vi "Acq FOR loop exit logic.vi"(8 "error in (no error)":errorcluster) -> (0 "error out (dupl)":errorcluster, 3 "Stop acquisition FOR loop":bool)   [LabVIEW 2013]
uses:
  Typedefs/Read Write Enum.ctl
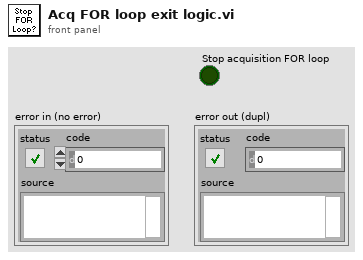
[diagram p1: front panel]
types:
  T1 = typedef "Read Write Enum.ctl" = enum16{"Read", "Write"}
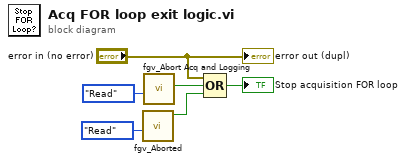
[diagram p0: block diagram]
diagram:
  n1 = call "fgv_Aborted.vi"("Function"=Read_Write_Enum."Read") -> ("Funct Acq Aborted?"=w1:bool)  [unwired: 9 in, 1 out]
  n2 = call "fgv_Abort Acq and Logging.vi"("Function"=Read_Write_Enum."Read") -> ("Abort acquisition"=w5:bool)  [unwired: 9 in, 1 out]
  n3 = Compound Arithmetic op=OR("error in (no error)", w5, w1) -> (→"Stop acquisition FOR loop":bool)
  "error out (dupl)" <- "error in (no error)"
